vi "New Pulse Acquired.vi"(8 "error in (no error)":errorcluster, 9 "Open plot":bool, 10 "Result in":refnum<class "Acquired Result.lvclass">, 11 "Monitor-Pulse in":refnum<class "LabActor.lvclass">) -> (0 "error out":errorcluster, 3 "Monitor-Pulse out":refnum<class "LabActor.lvclass">)   [LabVIEW 2018, in "LabActor.lvclass"]
uses:
  LabActor.lvclass
  NHMFL_Core/Libraries/Instruments/Results/Acquired Result/Acquired Result.lvclass
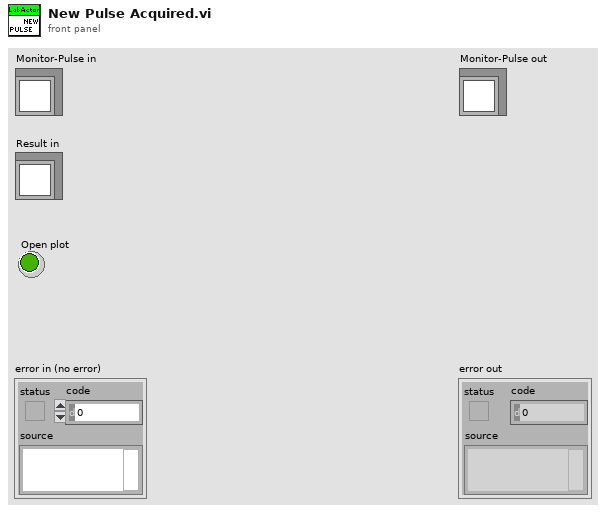
[diagram p1: front panel]
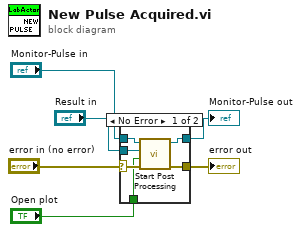
[diagram p0: block diagram]
diagram:
  n1 = case shown="No Error" "error in (no error)" {
    selector: "error in (no error)" -> [w12 w14]
    tunnel: [w8 w14] -> w5
    tunnel: [w9 w13] -> w3
    tunnel: "Monitor-Pulse in" -> [w11 w13]
    tunnel: "Result in" -> [w10 _]
    tunnel: "Open plot" -> [w7 _]
    frame No Error {
      n2 = call-dynamic "Start Post Processing.vi"("error in (no error)"=w12, "Open plot"=w7, "Result in"=w10, "Monitor-Pulse in"=w11) -> ("error out"=w8:errorcluster, "Monitor-Pulse out"=w9:refnum<class "LabActor.lvclass">)  [unwired: 5 in, 1 out]
    }
    frame Error {
    }
  }
  "error out" <- w5
  "Monitor-Pulse out" <- w3
